vi "NeuralNetwork.vi"() -> ()   [LabVIEW 2014]
panel:
  out "Array 2":dbl[](array[numeric])
  out "Array":dbl[](array[numeric])
  out "z":bool
  out "y":bool
  out "x":bool
  out "output wt":dbl[](array[numeric])
  out "hidden wt":dbl[](array[numeric])
  out "xyz":dbl[](array[numeric])
  in  "stop":bool
  in  "Training":bool
  out "Output":dbl[](array[numeric])
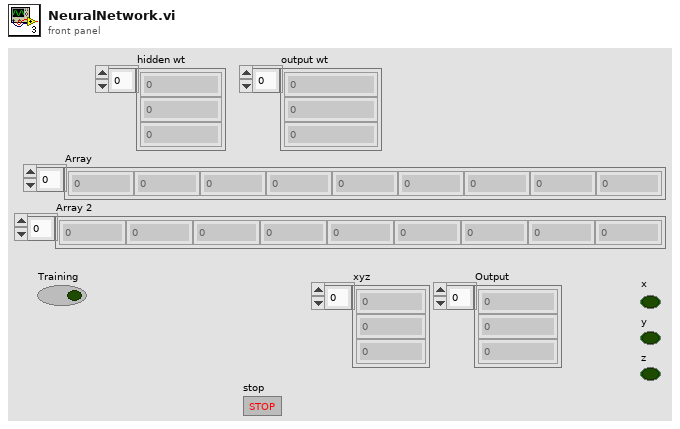
[diagram p1: front panel]
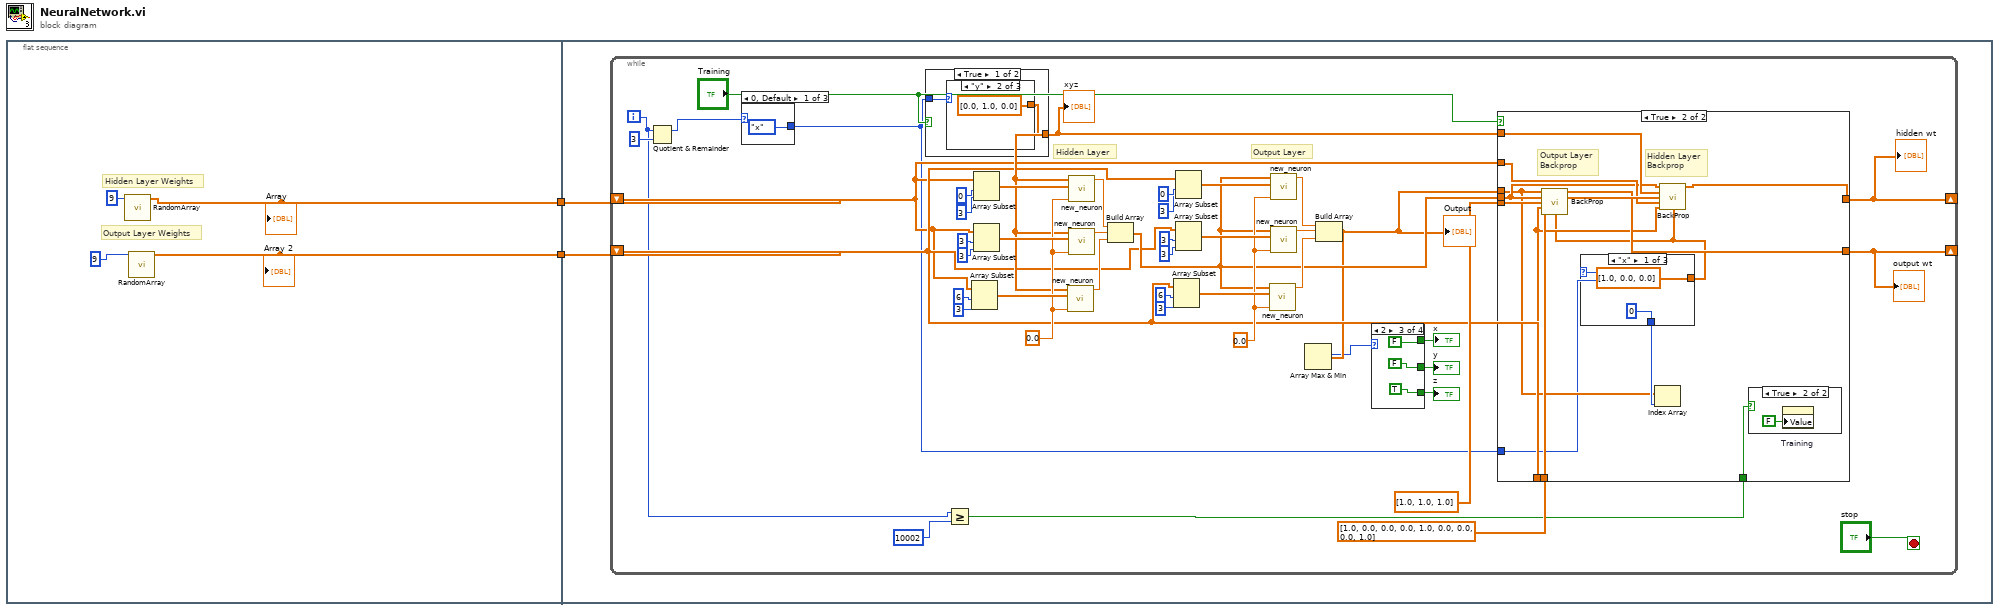
[diagram p0: block diagram]
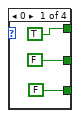
[diagram p2: hidden frame]
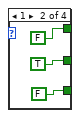
[diagram p3: hidden frame]
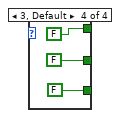
[diagram p4: hidden frame]
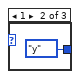
[diagram p5: hidden frame]
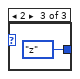
[diagram p6: hidden frame]
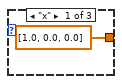
[diagram p7: hidden frame]
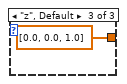
[diagram p8: hidden frame]
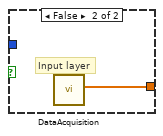
[diagram p9: hidden frame]
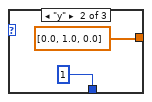
[diagram p12: hidden frame]
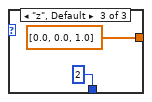
[diagram p13: hidden frame]
diagram:
  n1 = flat-sequence {
    tunnel: [w6] -> w2
    tunnel: [w5] -> w1
    tunnel: w2 -> [w8]
    tunnel: w1 -> [w7]
    frame #0 {
      # "Output Layer Weights"
      # "Hidden Layer Weights"
      n2 = call "RandomArray.vi"("Numeric"=9) -> ("Array"=w6:dbl[])  [unwired: 10 in]
      "Array" <- w6
      n3 = call "RandomArray.vi"("Numeric"=9) -> ("Array"=w5:dbl[])  [unwired: 10 in]
      "Array 2" <- w5
    }
    frame #1 {
      n4 = while {
        shift-right: [w25] -> _
        shift-left: w7 -> [w23]
        shift-right: [w21] -> _
        shift-left: w8 -> [w22]
        i -> [w11]
        stop <- "stop" stop-if-true
        w34 = 0.0 ("Offset")
        w46 = 0.0 ("Offset")
        # "Output Layer"
        # "Hidden Layer"
        n5 = Quotient & Remainder(x=w11, y=3) -> (x-y*floor(x/y)=w9:i32)  [unwired: 1 out]
        n6 = case shown="0, Default" w9 {
          tunnel: [enum16{"x", "y", "z"}."x" ("Enum") enum16{"x", "y", "z"}."y" ("Enum") enum16{"x", "y", "z"}."z" ("Enum")] -> w19
          frame 0, Default {
          }
          frame 1 {
          }
          frame 2 {
          }
        }
        n7 = case shown="True" "Training" {
          tunnel: [w71 w76] -> w29
          tunnel: w19 -> [w72 _]
          frame True {
            n8 = case shown="\"y\"" w72 {
              tunnel: [dbl[] [1.0, 0.0, 0.0] ("dE_dNET") dbl[] [0.0, 1.0, 0.0] ("dE_dNET") dbl[] [0.0, 0.0, 1.0] ("dE_dNET")] -> w71
              frame "x" {
              }
              frame "y" {
              }
              frame "z", Default {
              }
            }
          }
          frame False {
            # "Input layer"
            n9 = call "DataAcquisition.vi"() -> ("appended array"=w76:dbl[])  [unwired: 10 in, 1 out]
          }
        }
        "xyz" <- w29
        n10 = Greater Or Equal?(x=w11, y=10002) -> (x >= y?=w10:bool)
        n11 = Array Subset(array=w22, index=6, length=3) -> (w47:dbl[])
        n12 = Array Subset(array=w22, index=0, length=3) -> (w49:dbl[])
        n13 = Array Subset(array=w22, index=3, length=3) -> (w48:dbl[])
        n14 = call "new_neuron.vi"("Offset"=w46, "Weights"=w47, "Inputs"=w29) -> ("Output"=w35:dbl)  [unwired: 8 in]
        n15 = call "new_neuron.vi"("Offset"=w46, "Weights"=w49, "Inputs"=w29) -> ("Output"=w33:dbl)  [unwired: 8 in]
        n16 = call "new_neuron.vi"("Offset"=w46, "Weights"=w48, "Inputs"=w29) -> ("Output"=w36:dbl)  [unwired: 8 in]
        n17 = Build Array(w33, w36, w35) -> (w26:dbl[])
        n18 = Array Subset(array=w23, index=6, length=3) -> (w37:dbl[])
        n19 = Array Subset(array=w23, index=0, length=3) -> (w39:dbl[])
        n20 = Array Subset(array=w23, index=3, length=3) -> (w38:dbl[])
        n21 = call "new_neuron.vi"("Offset"=w34, "Weights"=w37, "Inputs"=w26) -> ("Output"=w30:dbl)  [unwired: 8 in]
        n22 = call "new_neuron.vi"("Offset"=w34, "Weights"=w39, "Inputs"=w26) -> ("Output"=w32:dbl)  [unwired: 8 in]
        n23 = call "new_neuron.vi"("Offset"=w34, "Weights"=w38, "Inputs"=w26) -> ("Output"=w31:dbl)  [unwired: 8 in]
        n24 = Build Array(w32, w31, w30) -> (w17:dbl[])
        "Output" <- w17
        n25 = Array Max & Min(array=w17) -> (max index (indices)=w13:i32)  [unwired: 3 out]
        n26 = case shown="2" w13 {
          tunnel: [TRUE FALSE FALSE FALSE] -> w16
          tunnel: [FALSE TRUE FALSE FALSE] -> w15
          tunnel: [FALSE FALSE TRUE FALSE] -> w14
          frame 0 {
          }
          frame 1 {
          }
          frame 2 {
          }
          frame 3, Default {
          }
        }
        "x" <- w16
        "y" <- w15
        "z" <- w14
        n27 = case shown="True" "Training" {
          tunnel: w22 -> [w78 w91]
          tunnel: w23 -> [w77 w85]
          tunnel: w29 -> [_ w90]
          tunnel: w17 -> [_ w81]
          tunnel: dbl[] [1.0, 1.0, 1.0] ("dE_dNET") -> [_ w89]
          tunnel: dbl[] [1.0, 0.0, 0.0, 0.0, 1.0, 0.0, 0.0, 0.0, 1.0] ("Target") -> [_ w88]
          tunnel: w26 -> [_ w83]
          tunnel: [w78 w87] -> w21
          tunnel: [w77 w86] -> w25
          tunnel: w19 -> [_ w80]
          tunnel: w10 -> [_ w79]
          frame False {
          }
          frame True {
            # "Hidden Layer\nBackprop"
            # "Output Layer\nBackprop"
            n28 = case shown="\"x\"" w80 {
              tunnel: [dbl[] [1.0, 0.0, 0.0] ("dE_dNET") dbl[] [0.0, 1.0, 0.0] ("dE_dNET") dbl[] [0.0, 0.0, 1.0] ("dE_dNET")] -> w84
              tunnel: [0 1 2] -> w82
              frame "x" {
              }
              frame "y" {
              }
              frame "z", Default {
              }
            }
            n29 = call "BackProp.vi"("Current Layer"=w81, "Previous Layer"=w83, "NetError"=w89, "weights"=w85, "PreviousWeights"=w88, "Target"=w84) -> ("w+"=w86:dbl[], "dE_dNET"=w92:dbl[])  [unwired: 8 in]
            n30 = Index Array(array=w81, index=w82) -> ()  [unwired: 1 out]
            n31 = call "BackProp.vi"("Current Layer"=w83, "Previous Layer"=w90, "NetError"=w92, "weights"=w91, "PreviousWeights"=w85, "Target"=w84) -> ("w+"=w87:dbl[])  [unwired: 8 in, 1 out]
            n32 = case shown="True" w79 {
              frame False {
              }
              frame True {
                n33 = property on="Training" class="Bool (strict)"("Value"=FALSE ("Training")) -> ()  [unwired: 2 in, 2 out]
              }
            }
          }
        }
        "hidden wt" <- w21
        "output wt" <- w25
      }
    }
  }
